vi "Check Last Write.vi"(8 "error in (no error)":errorcluster, 11 "Event Reporter Module in":refnum<class "Event Reporter Module.lvclass">) -> (0 "error out":errorcluster, 3 "Event Reporter Module out":refnum<class "Event Reporter Module.lvclass">)   [LabVIEW 2020, in "Volatus.lvlib" / "Event Reporter Module.lvclass"]
uses:
  Event Reporter Module.lvclass
  C:/dev/lv20CE/relink/lv-volatus/Volatus/Module/Module.lvclass
  Event Reporter Module.lvclass/Event Reporter Module.ctl
  Module/Module.lvclass/Module.ctl
  MessageQ/MessageQ.lvclass/MessageQ.ctl
  Module/Self Q.vi
  MessageQ/Send.vi
  Module/Module.lvclass
  C:/dev/lv20CE/relink/lv-volatus/Volatus/Event Reporter Module/Event Reporter Module.lvclass
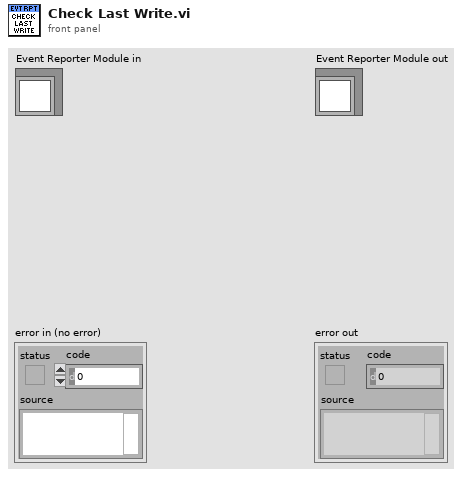
[diagram p1: front panel]
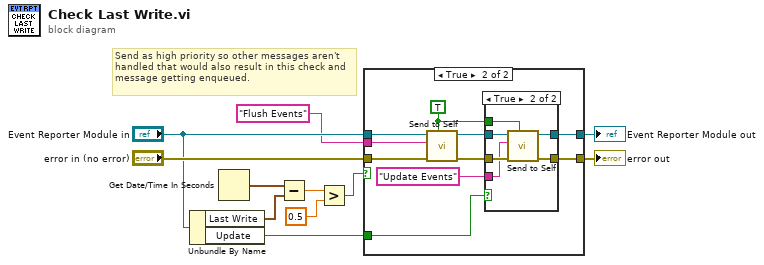
[diagram p0: block diagram]
diagram:
  # "Send as high priority so other messages aren't handled that would also result in this check and message getting enqueued."
  n1 = Unbundle By Name("Event Reporter Module in") -> ("Last Write"=w9:timestamp, "Update"=w1:bool)
  n2 = Get Date/Time In Seconds() -> (seconds since 1Jan1904=w10:timestamp)
  n3 = Subtract(x=w10, y=w9) -> (x-y=w8:dbl)
  n4 = Greater?(x=w8, y=0.5) -> (0:w2:bool)
  n5 = case shown="True" w2 {
    tunnel: "error in (no error)" -> [w13 w23]
    tunnel: [w13 w15] -> w6
    tunnel: "Event Reporter Module in" -> [w12 w22]
    tunnel: [w12 w16] -> w4
    tunnel: "Flush Events" ("Message ID") -> [_ w21]
    tunnel: w1 -> [_ w14]
    frame False {
    }
    frame True {
      w18 = TRUE ("High Priority (F)")
      n6 = call "Send to Self.vi"("High Priority (F)"=w18, "error in (no error)"=w23, "Message ID"=w21, "Module in"=w22) -> ("error out"=w19:errorcluster, "Module out"=w20:refnum<class "Event Reporter Module.lvclass">)  [unwired: 6 in]
      n7 = case shown="True" w14 {
        tunnel: w20 -> [w24 w31]
        tunnel: w19 -> [w25 w30]
        tunnel: w18 -> [_ w29]
        tunnel: "Update Events" ("Message ID") -> [_ w28]
        tunnel: [w24 w27] -> w16
        tunnel: [w25 w26] -> w15
        frame False {
        }
        frame True {
          n8 = call "Send to Self.vi"("High Priority (F)"=w29, "error in (no error)"=w30, "Message ID"=w28, "Module in"=w31) -> ("error out"=w26:errorcluster, "Module out"=w27:refnum<class "Event Reporter Module.lvclass">)  [unwired: 6 in]
        }
      }
    }
  }
  "error out" <- w6
  "Event Reporter Module out" <- w4
